vi "KG get reagent.vi"(8 "Fehler (Eingang, kein Fehler)":errorcluster, 10 "pump":u32, 11 "VISA-Ressourcenname":refnum<visa-resource-name>) -> (0 "Fehler (Ausgang)":errorcluster, 1 "Kommando gesendet":string, 2 "reagent":dbl, 3 "VISA-Ressourcenname (Ausgang)":refnum<visa-resource-name>)   [LabVIEW 2020, in "Linearisierung v2.lvlib" / "Gasteiler.lvlib" / "HovaCAL_Interface.lvlib" / "KGN.lvlib" / "get.lvlib"]
uses:
  get.lvlib
  KGN.lvlib
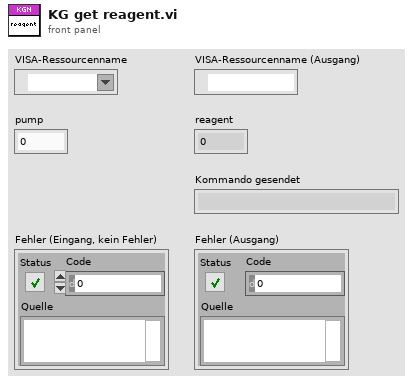
[diagram p1: front panel]
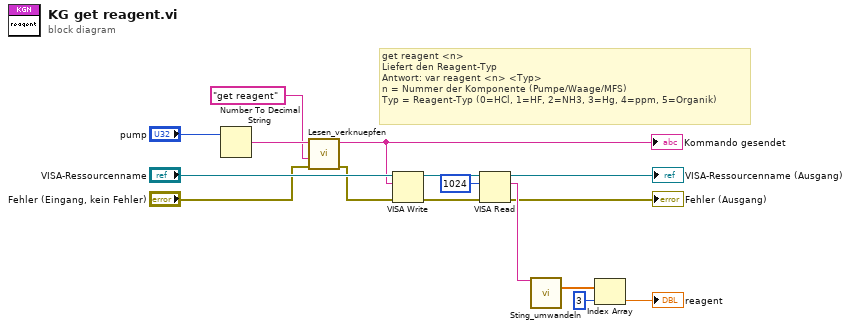
[diagram p0: block diagram]
diagram:
  # "get reagent <n>\nLiefert den Reagent-Typ\nAntwort: var reagent <n> <Typ>\nn = Nummer der Komponente (Pumpe/Waage/MFS)\nTyp = Reagent-Typ (0=HCl, 1=HF, 2=NH3, 3=Hg, 4=ppm, 5=Organik)"
  n1 = Number To Decimal String(number="pump") -> (decimal integer string=w5:string)  [unwired: 1 in]
  n2 = call "Lesen_verknuepfen.vi"("error in (no error)"="Fehler (Eingang, kein Fehler)", "Order"="get reagent" ("Schreibpuffer"), "param"=w5) -> ("error out"=w7:errorcluster, "Verknüpfter String"=w6:string)  [unwired: 7 in]
  "Kommando gesendet" <- w6
  n3 = VISA Write(VISA resource name="VISA-Ressourcenname", write buffer=w6, error in (no error)=w7) -> (VISA resource name out=w16:refnum<visa-resource-name>, error out=w15:errorcluster)  [unwired: 1 out]
  n4 = VISA Read(VISA resource name=w16, byte count=u32 1024 ("Byte-Anzahl"), error in (no error)=w15) -> (VISA resource name out=→"VISA-Ressourcenname (Ausgang)":refnum<visa-resource-name>, read buffer=w13:string, error out=→"Fehler (Ausgang)":errorcluster)  [unwired: 1 out]
  n5 = call "Sting_umwandeln.vi"("Lesepuffer"=w13) -> ("Zahl array"=w2:dbl[])  [unwired: 8 in, 6 out]
  n6 = Index Array(array=w2, index=3 ("Index")) -> (element=→"reagent":dbl)
